vi "LCR_Readout.vi"(8 "error in (no error)":errorcluster, 10 "Frequency in Hz":i32, 11 "HP4284 in":refnum<class "HP4284.lvclass">) -> (0 "error out":errorcluster, 1 "Resistance in MOhm":dbl, 2 "Capacitance in pF":dbl, 3 "HP4284 out":refnum<class "HP4284.lvclass">)   [LabVIEW 2018, in "HP4284.lvclass"]
uses:
  HP4284.lvclass
panel:
  out "Data status":i32
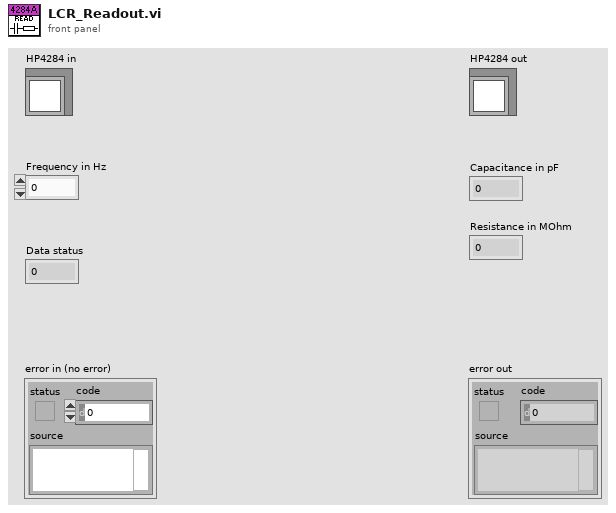
[diagram p1: front panel]
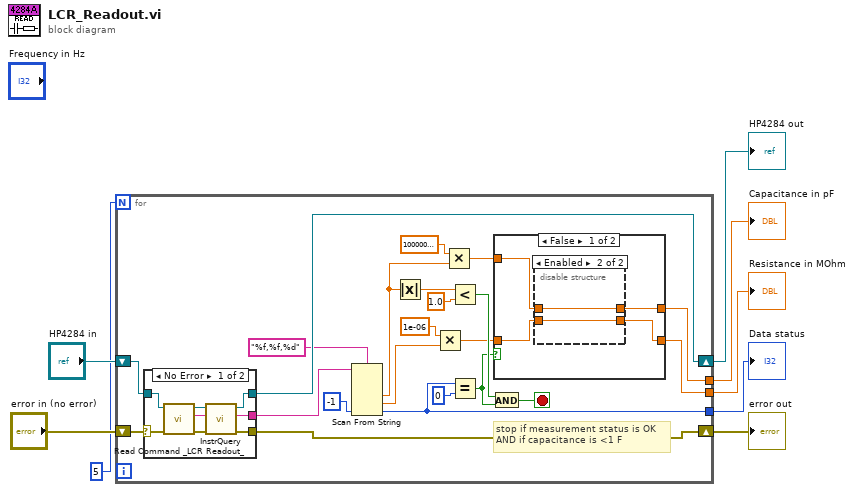
[diagram p0: block diagram]
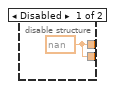
[diagram p2: hidden frame]
diagram:
  n1 = for {
    N: 5 -> [_]
    tunnel: [w16] -> w4
    tunnel: [w13] -> w3
    tunnel: [w11] -> w2
    shift-right: [w29] -> w7
    shift-left: "HP4284 in" -> [w30]
    shift-right: [w28] -> w6
    shift-left: "error in (no error)" -> [w27]
    stop <- w14 stop-if-true
    # "stop if measurement status is OK\nAND if capacitance is <1 F"
    n2 = case shown="No Error" w27 {
      selector: w27 -> [w41 w48]
      tunnel: w30 -> [w47 w49]
      tunnel: [w43 w49] -> w29
      tunnel: [w42 w48] -> w28
      tunnel: [w40 _] -> w24
      frame No Error {
        n3 = call-dynamic "Read Command _LCR Readout_.vi"("error in (no error)"=w41, "LCRControl in"=w47) -> ("error out"=w44:errorcluster, "Command \"LCR Readout\""=w45:string, "LCRControl out"=w46:refnum<class "HP4284.lvclass">)  [unwired: 7 in]
        n4 = call-dynamic "InstrQuery.vi"("error in (no error)"=w44, "Command string"=w45, "InstControl in"=w46) -> ("error out"=w42:errorcluster, "Instrument response"=w40:string, "InstControl out"=w43:refnum<class "HP4284.lvclass">)  [unwired: 6 in]
      }
      frame Error {
      }
    }
    n5 = Scan From String(format string="%f,%f,%d", input string=w24, default 3=-1 ("default value 3")) -> (output 1=w20:dbl, output 2=w22:dbl, output 3=w16:i32)  [unwired: 4 in, 3 out]
    n6 = Absolute Value(x=w20) -> (abs(x)=w19:dbl)
    n7 = Multiply(x=1e-06, y=w22) -> (x*y=w9:dbl)
    n8 = Multiply(x=1000000000000.0, y=w20) -> (x*y=w12:dbl)
    n9 = Less?(x=w19, y=1.0) -> (x < y?=w17:bool)
    n10 = Equal?(x=w16, y=0) -> (x = y?=w10:bool)
    n11 = And(x=w17, y=w10) -> (x .and. y?=w14:bool)
    n12 = case shown="False" w10 {
      tunnel: [w33 w39] -> w13
      tunnel: w12 -> [w34 w39]
      tunnel: [w31 w38] -> w11
      tunnel: w9 -> [w32 w38]
      frame False {
        n13 = disable-structure shown="Enabled" {
          disable-tunnel: [w35 w36] -> w31
          disable-tunnel: w34 -> [_ w37]
          disable-tunnel: [w35 w37] -> w33
          disable-tunnel: w32 -> [_ w36]
          frame Disabled {
            w35 = nan
          }
          frame Enabled {
          }
        }
      }
      frame True {
      }
    }
  }
  "error out" <- w6
  "HP4284 out" <- w7
  "Capacitance in pF" <- w3
  "Resistance in MOhm" <- w2
  "Data status" <- w4
